vi "Get AccessSDO.vi"(8 "Error In":errorcluster, 11 "reference in":refnum<class "OD Sub-Entry.lvclass">) -> (0 "Error Out":errorcluster, 2 "Access SDO":T1, 3 "reference out":refnum<class "OD Sub-Entry.lvclass">)   [LabVIEW 2019, in "Electronic Datasheet.lvlib" / "OD Sub-Entry.lvclass"]
uses:
  OD Sub-Entry.lvclass
  OD Entry/OD Entry.lvclass
  Object Type.ctl
  Electronic Datasheet.lvlib
  Access SDO.ctl
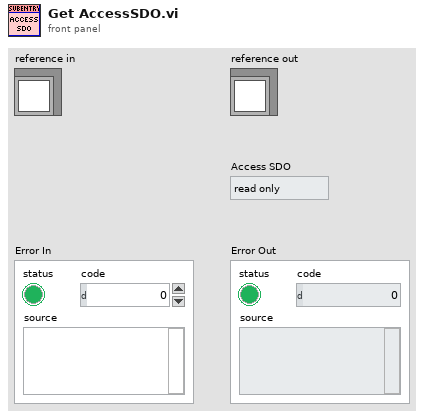
[diagram p1: front panel]
types:
  T1 = typedef "Electronic Datasheet.lvlib/Access SDO.ctl" = enum16{"read only", "write only", "read/write", "read/write on process input", "read/write on process output", "constant value", "no", "UNKNOWN"}
  T2 = enum16{"ro", "wo", "rw", "rwr", "rww", "const", "UNKNOWN"}
  T3 = typedef "Electronic Datasheet.lvlib/Object Type.ctl" = u8
  T4 = typedef "Electronic Datasheet.lvlib/OD Sub-Entry.lvclass/ObjectAttributes.ctl" = cluster{"Parent":refnum<class "OD Entry.lvclass">}
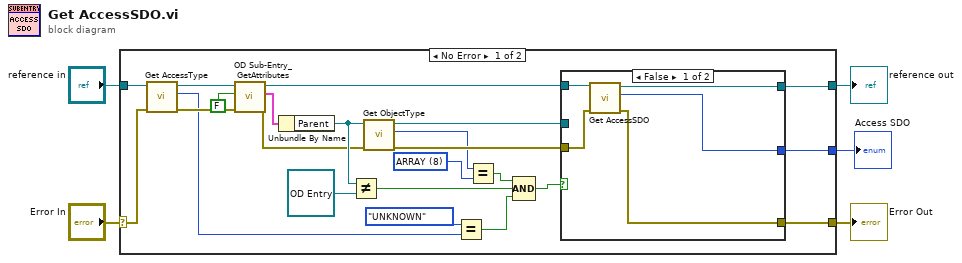
[diagram p0: block diagram]
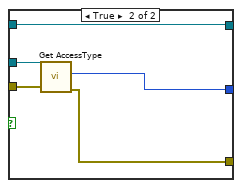
[diagram p2: hidden frame]
diagram:
  n1 = case shown="No Error" "Error In" {
    selector: "Error In" -> [w28 w40]
    tunnel: [w27 w40] -> w4
    tunnel: [w12 w39] -> w2
    tunnel: "reference in" -> [w10 w39]
    tunnel: [w14 _] -> w1
    frame No Error {
      w17 = T3 8 items=["NULL"=0, "DOMAIN"=2, "DEFTYPE"=5, "DEFSTRUCT"=6, "VAR"=7, "ARRAY"=8, "RECORD"=9] ("ObjectType")
      n2 = call "Get AccessType.vi"("Error In"=w28, "reference in"=w10) -> ("Error Out"=w11:errorcluster, "AccessType"=w7:T2, "reference out"=w9:refnum<class "OD Sub-Entry.lvclass">)  [unwired: 7 in]
      n3 = call "OD Sub-Entry_GetAttributes.vi"("Error In"=w11, "OnlyGetDvrReference(False)"=FALSE, "reference in"=w9) -> ("Error Out"=w20:errorcluster, "Data"=w25:T4, "reference out"=w13:refnum<class "OD Sub-Entry.lvclass">)  [unwired: 5 in, 1 out]
      n4 = Unbundle By Name(w25) -> ("Parent"=w21:refnum<class "OD Entry.lvclass">)
      n5 = Not Equal?(x=w21, y=refnum<class "OD Entry.lvclass"> refnum ("Electronic Datasheet.lvlib:OD Entry")) -> (x != y?=w23:bool)
      n6 = call "Get ObjectType.vi"("Error In"=w20, "reference in"=w21) -> ("Error Out"=w19:errorcluster, "ObjectType"=w16:T3, "reference out"=w15:refnum<class "OD Entry.lvclass">)  [unwired: 7 in]
      n7 = Equal?(x=T2."UNKNOWN", y=w7) -> (x = y?=w8:bool)
      n8 = Equal?(x=w16, y=w17) -> (x = y?=w18:bool)
      n9 = Compound Arithmetic op=AND(w18, w23, w8) -> (w22:bool)
      n10 = case shown="False" w22 {
        tunnel: [w31 w36] -> w27
        tunnel: w19 -> [w32 w37]
        tunnel: w15 -> [_ w38]
        tunnel: [w30 w35] -> w14
        tunnel: w13 -> [w33 w34]
        tunnel: [w29 w34] -> w12
        frame False {
          n11 = call-parent "Get AccessSDO.vi"("error in"=w32, "OD Entry in"=w33) -> ("error out"=w31:errorcluster, "Access SDO"=w30:T1, "OD Entry out"=w29:refnum<class "OD Sub-Entry.lvclass">)  [unwired: 7 in]
        }
        frame True {
          n12 = call "Get AccessType.vi"("Error In"=w37, "reference in"=w38) -> ("Error Out"=w36:errorcluster, "AccessType"=w35:T2)  [unwired: 7 in, 1 out]
        }
      }
    }
    frame Error {
    }
  }
  "Error Out" <- w4
  "reference out" <- w2
  "Access SDO" <- w1
